vi "SpectrometerTestGPIO.vi"() -> ()   [LabVIEW 2015]
panel:
  in  "AUX Value":bool
  out "Total\nGPIO Bits":i32=6
  in  "direction bit":bool=TRUE
  out "Number of Pins":i32=6
  in  "Value":bool
  out "Spectrum of the first Spectrometer":cluster{"Y":dbl[], "Y":dbl[]}[](graph)
  in  "stop":bool
  in  "Enter the \nInetegration Time":i32
  in  "Start":bool
  out "Number of Spectrometers":i32=1
  # "GPIO Pin 0"
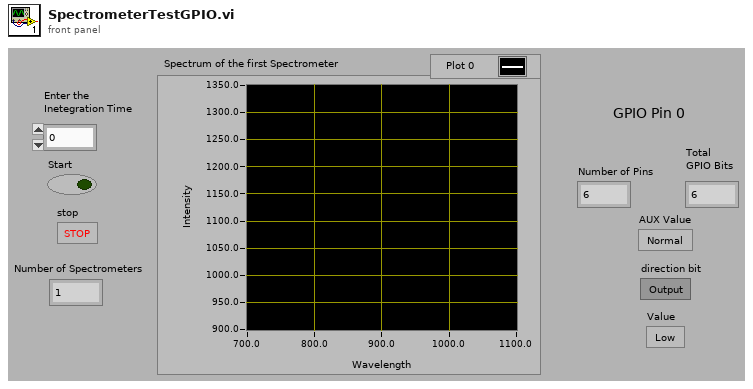
[diagram p1: front panel]
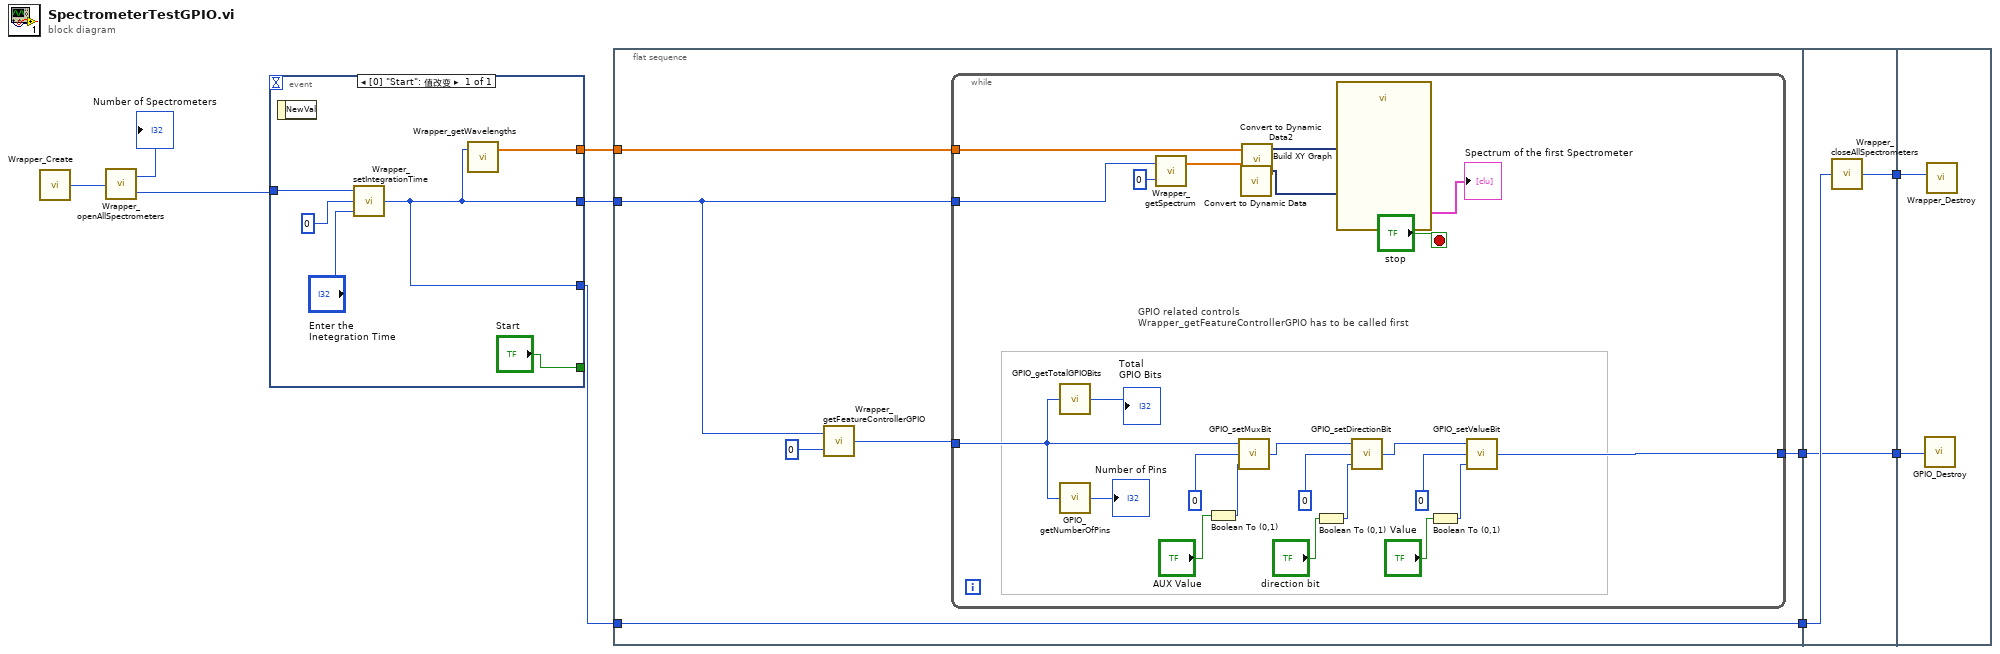
[diagram p0: block diagram]
diagram:
  n1 = call "Wrapper_Create.vi"() -> ("Wrapper"=w10:u32)
  n2 = call "Wrapper_openAllSpectrometers.vi"("Wrapper In"=w10) -> ("Number of Spectrometers"=→"Number of Spectrometers":i32, "Wrapper Out"=w8:u32)
  n3 = event shown="[0] \"Start\": 值改变" {
    selector: _ -> [_]
    dyn-events: _ -> [_]
    timeout: _ -> [_]
    tunnel: ["Start"] -> _
    tunnel: w8 -> [w13]
    tunnel: [w11] -> w7
    tunnel: [w12] -> w6
    tunnel: [w11] -> w4
    event "Start": Value Change {
      n4 = event-data() -> ()  [unwired: 1 in, 1 out]
      n5 = call "Wrapper_setIntegrationTime.vi"("Integration Time"="Enter the \nInetegration Time", "Index"=0, "Wrapper In"=w13) -> ("Wrapper Out"=w11:u32)
      n6 = call "Wrapper_getWavelengths.vi"("Wrapper"=w11) -> ("WL Values"=w12:dbl[])  [unwired: 1 in, 1 out]
    }
  }
  n7 = flat-sequence {
    tunnel: w7 -> [w18]
    tunnel: w6 -> [w22]
    tunnel: [w21] -> w5
    tunnel: w4 -> [w21]
    tunnel: [w20] -> w1
    tunnel: w5 -> [w48]
    tunnel: [w47] -> w3
    tunnel: [w46] -> w2
    tunnel: w1 -> [w46]
    tunnel: w3 -> [w50]
    tunnel: w2 -> [w49]
    frame #0 {
      n8 = call "Wrapper_getFeatureControllerGPIO.vi"("Index"=0, "Wrapper"=w18) -> ("GPIO"=w17:u32)
      n9 = while {
        tunnel: w18 -> [w37]
        tunnel: w22 -> [w40]
        tunnel: [w38] -> w20
        tunnel: w17 -> [w30]
        stop <- "stop" stop-if-true
        # "GPIO related controls\nWrapper_getFeatureControllerGPIO has to be called first"
        n10 = call "GPIO_getTotalGPIOBits.vi"("GPIO"=w30) -> ("Total\nGPIO Bits"=→"Total\nGPIO Bits":i32)
        n11 = call "GPIO_getNumberOfPins.vi"("GPIO"=w30) -> ("Number of Pins"=→"Number of Pins":i32)
        n12 = call "Wrapper_getSpectrum.vi"("Index"=0, "Wrapper"=w37) -> ("Spectrum Values"=w42:dbl[])  [unwired: 1 out]
        n13 = Boolean To (0,1)(Boolean="AUX Value") -> (0, 1=w27:i16)
        n14 = call "GPIO_setMuxBit.vi"("Bit Value"=w27, "Bit Number"=0, "GPIO In"=w30) -> ("GPIO Out"=w29:u32)
        n15 = call "Convert to Dynamic Data"("Array"=w42) -> ("Dynamic Data Type"=w41:dynamicdata)  [unwired: 3 in]
        n16 = call "Convert to Dynamic Data2"("Array"=w40) -> ("Dynamic Data Type"=w39:dynamicdata)  [unwired: 3 in]
        n17 = Boolean To (0,1)(Boolean="direction bit") -> (0, 1=w26:i16)
        n18 = call "Build XY Graph"("Y Input"=w41, "X Input"=w39) -> ("XY Graph"=→"Spectrum of the first Spectrometer":cluster{"Y":dbl[], "Y":dbl[]}[])  [unwired: 8 in, 1 out]
        n19 = call "GPIO_setDirectionBit.vi"("Value"=w26, "Bit"=0, "GPIO In"=w29) -> ("GPIO Out"=w33:u32)
        n20 = Boolean To (0,1)(Boolean="Value") -> (0, 1=w25:i16)
        n21 = call "GPIO_setValueBit.vi"("Value"=w25, "Bit"=0, "GPIO In"=w33) -> ("GPIO Out"=w38:u32)
      }
    }
    frame #1 {
      n22 = call "Wrapper_closeAllSpectrometers.vi"("Wrapper In"=w48) -> ("Wrapper Out"=w47:u32)
    }
    frame #2 {
      n23 = call "GPIO_Destroy.vi"("GPIO"=w49) -> ()
      n24 = call "Wrapper_Destroy.vi"("Wrapper"=w50) -> ()
    }
  }
